vi "Template Add.vi"(8 "error in (no error)":errorcluster, 9 "Parameters (empty)":T1, 10 "Template Record":T2, 11 "Connection Refnum":T3) -> (0 "error out":errorcluster, 2 "New Template Record":T2, 3 "Connection Refnum":T3)   [LabVIEW 2011]
uses:
  Template Record.ctl
  SI.LIB/ODBC/SQL Controls/Connection Refnum.ctl
  Addons/internet/utils/keyedarr.llb/Keyed Array.ctl
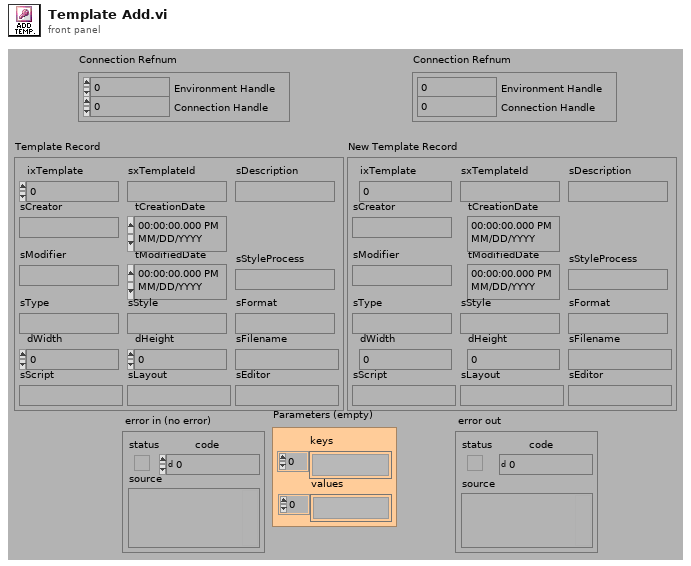
[diagram p1: front panel]
types:
  T1 = typedef "Keyed Array.ctl" = cluster{"keys":string[], "values":string[]}
  T2 = typedef "Template Record.ctl" = cluster{"ixTemplate":i32, "sxTemplateId":string, "sDescription":string, "sCreator":string, "tCreationDate":timestamp, "sModifier":string, "tModifiedDate":timestamp, "sType":string, "sStyle":string, "sFormat":string, "dWidth":dbl, "dHeight":dbl, "sFilename":string, "sScript":string, "sLayout":string, "sEditor":string, "sStyleProcess":string}
  T3 = typedef "Connection Refnum.ctl" = cluster{"Environment Handle":i32, "Connection Handle":i32}
  T4 = typedef "Statement Refnum.ctl" = cluster{"Statement Handle":i32, "Parameter Number":u16}
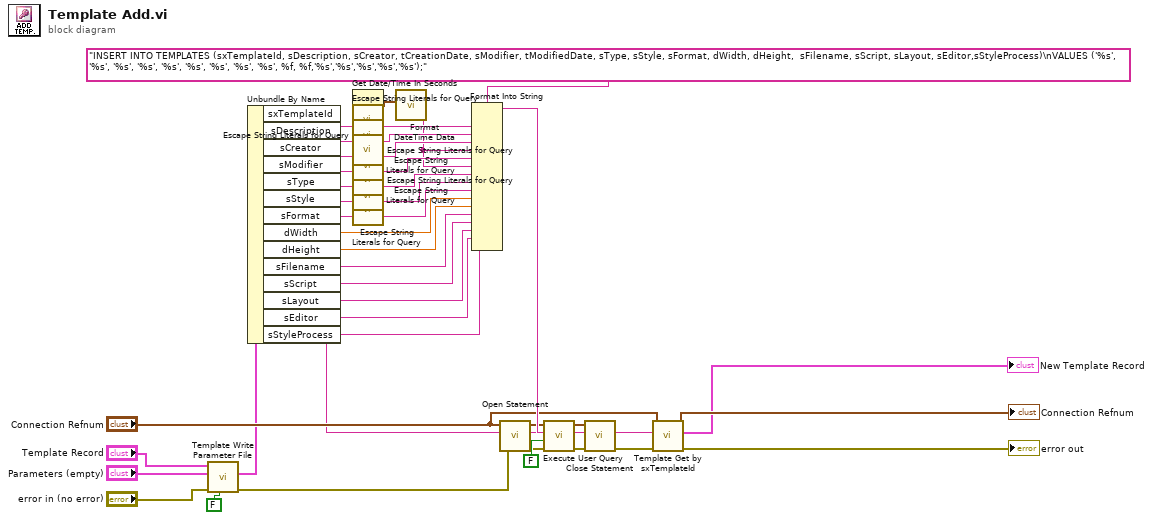
[diagram p0: block diagram]
diagram:
  n1 = call "Template Write Parameter File.vi"("Export?"=FALSE ("Load Content for export?"), "error in (no error)"="error in (no error)", "Parameters (empty)"="Parameters (empty)", "Template Record"="Template Record") -> ("error out"=w4:errorcluster, "Template Record 2"=w3:T2)  [unwired: 2 in, 4 out]
  n2 = Unbundle By Name(w3) -> ("sxTemplateId"=w6:string, "sDescription"=w33:string, "sCreator"=w32:string, "sModifier"=w30:string, "sType"=w28:string, "sStyle"=w27:string, "sFormat"=w21:string, "dWidth"=w24:dbl, "dHeight"=w23:dbl, "sFilename"=w15:string, "sScript"=w14:string, "sLayout"=w13:string, "sEditor"=w12:string, "sStyleProcess"=w1:string)
  n3 = Get Date/Time In Seconds() -> (seconds since 1Jan1904=w25:timestamp)
  n4 = call "Escape String Literals for Query.vi"("String"=w6) -> ("escaped String"=w18:string)  [unwired: 1 in, 13 out]
  n5 = call "Escape String Literals for Query.vi"("String"=w33) -> ("escaped String"=w34:string)  [unwired: 1 in, 13 out]
  n6 = call "Escape String Literals for Query.vi"("String"=w32) -> ("escaped String"=w31:string)  [unwired: 1 in, 13 out]
  n7 = call "Escape String Literals for Query.vi"("String"=w30) -> ("escaped String"=w29:string)  [unwired: 1 in, 13 out]
  n8 = call "Escape String Literals for Query.vi"("String"=w28) -> ("escaped String"=w19:string)  [unwired: 1 in, 13 out]
  n9 = call "Escape String Literals for Query.vi"("String"=w27) -> ("escaped String"=w22:string)  [unwired: 1 in, 13 out]
  n10 = call "Escape String Literals for Query.vi"("String"=w21) -> ("escaped String"=w20:string)  [unwired: 1 in, 13 out]
  n11 = call "Format DateTime Data.vi"("Timestamp in"=w25) -> ("UTC DB String out"=w17:string)  [unwired: 10 out]
  n12 = Format Into String(format string="INSERT INTO TEMPLATES (sxTemplateId, sDescription, sCreator, tCreationDate, sModifier, tModifiedDate, sType, sStyle, sFormat, dWidth, dHeight,  sFilename, sScript, sLayout, sEditor,sStyleProcess)\nVALUES ('%s', '%s', '%s', '%s', '%s', '%s', '%s', '%s', '%s', %f, %f,'%s','%s','%s','%s','%s');" ("User Query"), w18, w34, w31, w17, w29, w17, w19, w22, w20, w24, w23, w15, w14, w13, w12, w1) -> (resulting string=w40:string)  [unwired: 2 in, 1 out]
  n13 = call "Open Statement.vi"("error in (no error)"=w4, "Connection Refnum"="Connection Refnum") -> ("error out"=w36:errorcluster, "Statement Refnum"=w35:T4)  [unwired: 4 out]
  n14 = call "Execute User Query.vi"("error in (no error)"=w36, "Return Data? (f)"=FALSE, "User Query"=w40, "Statement Refnum"=w35) -> ("error out"=w37:errorcluster, "Statement Refnum"=w38:T4)  [unwired: 2 out]
  n15 = call "Close Statement.vi"("error in (no error)"=w37, "Statement Refnum"=w38) -> ("error out"=w2:errorcluster)  [unwired: 5 out]
  n16 = call "Template Get by sxTemplateId.vi"("error in (no error)"=w2, "sxTemplateId (\"\")"=w6, "Connection Refnum"="Connection Refnum") -> ("error out"=→"error out":errorcluster, "Template Record"=→"New Template Record":T2, "Connection Refnum"=→"Connection Refnum":T3)  [unwired: 6 out]
